vi "AAL Resample (Const to Variable).vi"(7 "reset? (True)":bool=TRUE, 8 "error in (no error)":errorcluster, 9 "config":T1={"timing jitter"=enum."Interpolation", "anti-aliasing?"=TRUE, "filter prototype"={"coefficients"=[], "factor"=1}} {"filter prototype"."coefficients" format="%.2f"}, 10 "time":dbl[](array[numeric]) format="%.2f", 11 "X":dbl[](array[numeric])) -> (0 "error out":errorcluster, 1 "offset":i64, 2 "time stamps":dbl[](array[numeric]) format="%.2f", 3 "Y":dbl[](array[numeric]) format="%.2f")   [LabVIEW 2017, in "NI_AALPro.lvlib"]
doc: "Perform an arbitrary resampling on the input signal."
uses:
  NI_AALPro.lvlib
  lvanlys.dll
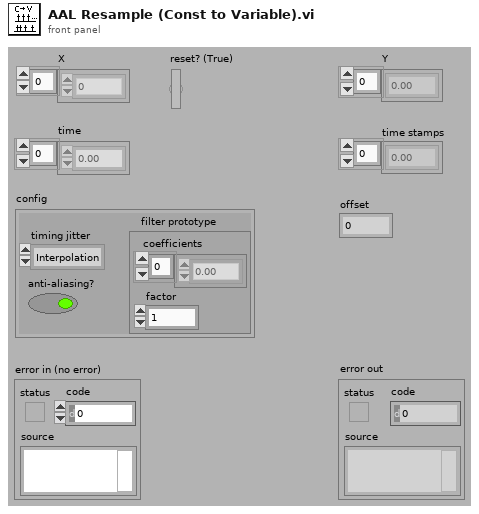
[diagram p1: front panel]
types:
  T1 = cluster{"timing jitter":enum32{"Interpolation", "Rounding"}, "anti-aliasing?":bool, "filter prototype":cluster{"coefficients":dbl[], "factor":i32}}
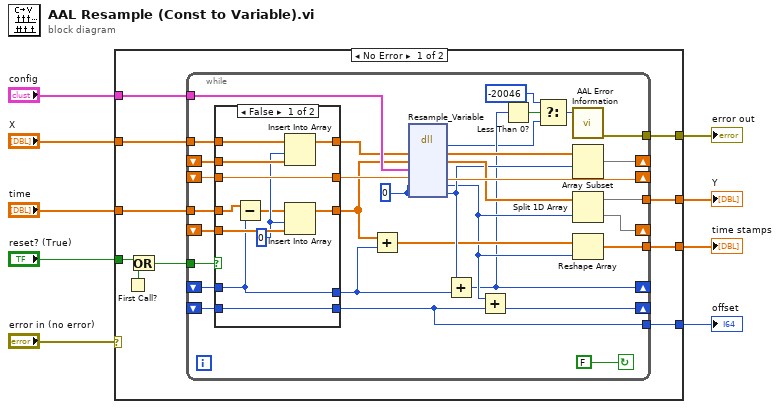
[diagram p0: block diagram]
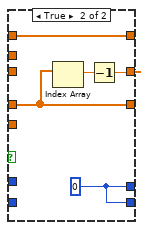
[diagram p2: hidden frame]
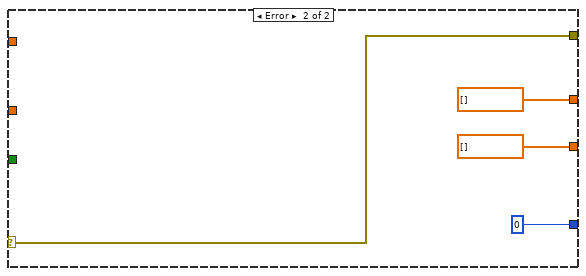
[diagram p3: hidden frame]
diagram:
  n1 = case shown="No Error" "error in (no error)" {
    selector: "error in (no error)" -> [_ w72]
    tunnel: "config" -> [w18 _]
    tunnel: "reset? (True)" -> [w17 _]
    tunnel: "time" -> [w11 _]
    tunnel: [w15 dbl[] []] -> w6
    tunnel: [w14 dbl[] []] -> w5
    tunnel: [w13 i64 0] -> w4
    tunnel: [w12 w72] -> w3
    tunnel: "X" -> [w10 _]
    frame No Error {
      n2 = First Call?() -> (First Call?: T/F=w19:bool)
      n3 = Or(x=w17, y=w19) -> (x .or. y?=w16:bool)
      n4 = while {
        tunnel: [w37] -> w14
        tunnel: [w25] -> w15
        shift-right: [w50] -> _
        shift-left: _ -> [w42]
        shift-right: [w51] -> _
        shift-left: _ -> [w43]
        tunnel: w10 -> [w47]
        tunnel: w11 -> [w45]
        shift-right: [w49] -> _
        shift-left: _ -> [w41]
        tunnel: w16 -> [w40]
        tunnel: w18 -> [w52]
        shift-right: [w24] -> _
        shift-left: _ -> [w38]
        tunnel: [w28] -> w13
        shift-right: [w27] -> _
        shift-left: _ -> [w31]
        tunnel: [w26] -> w12
        stop <- FALSE continue-if-true
        w33 = 0
        n5 = case shown="False" w40 {
          tunnel: [w62 w68] -> w46
          tunnel: w47 -> [w60 w68]
          tunnel: [w57 w67] -> w35
          tunnel: w45 -> [w56 w67]
          tunnel: [w63 w65] -> w44
          tunnel: w43 -> [w59 _]
          tunnel: w42 -> [w61 _]
          tunnel: w41 -> [w63 _]
          tunnel: w38 -> [w54 _]
          tunnel: [w54 w64] -> w29
          tunnel: w31 -> [w53 _]
          tunnel: [w53 w64] -> w28
          frame False {
            w58 = 0 ("Index")
            n6 = Subtract(x=w56, y=w54) -> (x-y=w55:dbl[])
            n7 = Insert Into Array(array=w60, index=w58, new element=w59) -> (w62:dbl[])
            n8 = Insert Into Array(array=w55, index=w58, new element=w61) -> (w57:dbl[])
          }
          frame True {
            w64 = i64 0
            n9 = Index Array(array=w67) -> (element=w66:dbl)  [unwired: 1 in]
            n10 = Decrement(x=w66) -> (x-1=w65:dbl)
          }
        }
        n11 = Add(x=w35, y=w29) -> (x+y=w34:dbl[])
        n12 = dll-call lib="C:/Program Files/National Instruments/LabVIEW 2017/resource/lvanlys.*" fn="Resample_Variable"("xH"=w46, "timeH"=w35, "config"=w52, "last_sample_time"=w44, "out_len"=w33, "xLeftOverIdx"=w33) -> (w22:i32, "xH"=w32:dbl[], "timeH"=w39:dbl[], "last_sample_time"=w49:dbl, "out_len"=w30:i32, "xLeftOverIdx"=w36:i32)  [unwired: 4 in, 2 out]
        n13 = Add(x=w36, y=w29) -> (x+y=w24:i64)
        n14 = Add(x=w30, y=w28) -> (x+y=w27:i64)
        n15 = Less Than 0?(x=w24) -> (x < 0?=w23:bool)
        n16 = Select(t=-20046 ("error"), s=w23, f=w22) -> (s? t:f=w20:i32)
        n17 = call "AAL Error Information.vi"("error code"=w20) -> ("error out"=w26:errorcluster)  [unwired: 10 in]
        n18 = Array Subset(array=w32, index=w36) -> (w51:dbl[])  [unwired: 1 in]
        n19 = Split 1D Array(array=w39, index=w30) -> (first subarray=w37:dbl[], second subarray=w50:dbl[])
        n20 = Reshape Array(w34, w30) -> (w25:dbl[])
      }
    }
    frame Error {
    }
  }
  "time stamps" <- w6
  "Y" <- w5
  "offset" <- w4
  "error out" <- w3
